vi "TestTarget2.vi"(8 "Error In":errorcluster, 11 "Top-Left":string) -> (0 "Error Out":errorcluster, 3 "Top-Right":string)   [LabVIEW 2014, in "TestVIs.lvlib"]
uses:
  TestVIs.lvlib
panel:
  in  "File Path Control":path
  in  "Control-Num 3":dbl
  in  "Control-Num 2":dbl
  in  "Control-Num 1":dbl
  in  "Control-String 2":string
  in  "Control-String 1":string
  in  "Cancel Button":bool
  in  "OK Button":bool
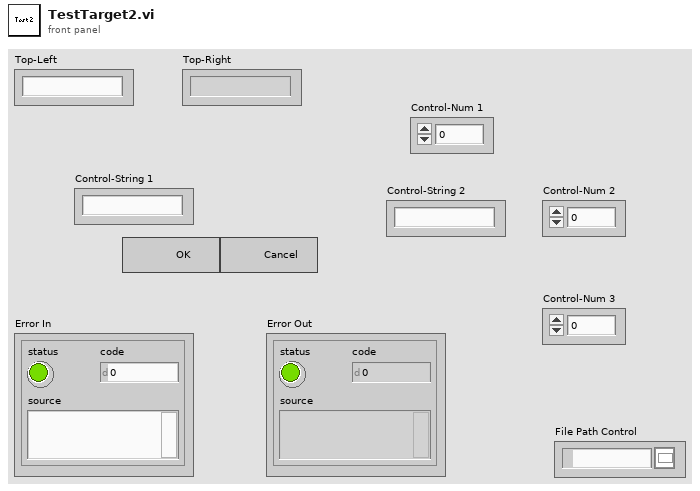
[diagram p1: front panel]
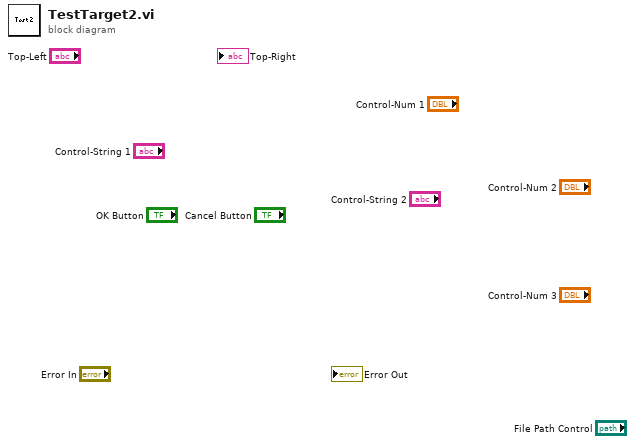
[diagram p0: block diagram]
diagram:
